vi "Decrement Counter.vi"(5 "Tag Values":string[](array[string]), 7 "Tags":string[](array[string]), 8 "error in (no error)":errorcluster, 9 "Value (1)":i32=1, 10 "Metric Name":string, 11 "StatD Interface in":refnum<class "StatD Interface.lvclass">) -> (0 "error out":errorcluster, 3 "StatD Interface out":refnum<class "StatD Interface.lvclass">)   [LabVIEW 2011, in "StatD Interface.lvclass"]
doc: "Decrement a counter by the amount specified in value (default 1)."
uses:
  StatD Interface.lvclass
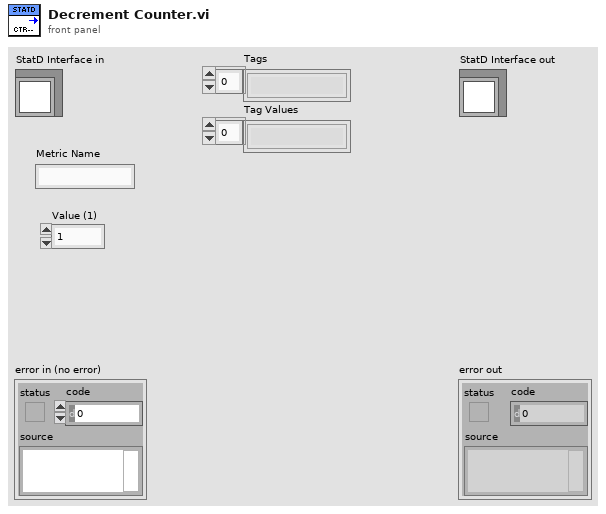
[diagram p1: front panel]
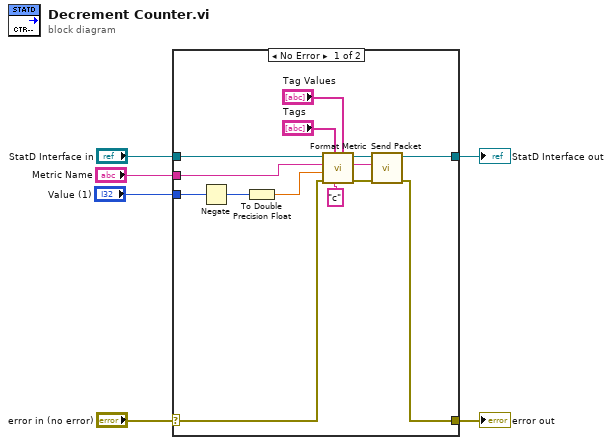
[diagram p0: block diagram]
diagram:
  n1 = case shown="No Error" "error in (no error)" {
    selector: "error in (no error)" -> [w9 w22]
    tunnel: [w19 w22] -> w5
    tunnel: [w20 w21] -> w3
    tunnel: "StatD Interface in" -> [w15 w21]
    tunnel: "Value (1)" -> [w11 _]
    tunnel: "Metric Name" -> [w10 _]
    frame No Error {
      n2 = Negate(x=w11) -> (-x=w7:i32)
      n3 = To Double Precision Float(number=w7) -> (double precision float=w8:dbl)
      n4 = call "Format Metric.vi"("Tag Values"="Tag Values", "Metric Type"="c", "Tags"="Tags", "error in (no error)"=w9, "Metric Value"=w8, "Metric Name"=w10, "StatD Interface in"=w15) -> ("error out"=w17:errorcluster, "Packet"=w16:string, "StatD Interface out"=w18:refnum<class "StatD Interface.lvclass">)  [unwired: 2 in]
      n5 = call "Send Packet.vi"("error in (no error)"=w17, "Packet"=w16, "StatD Interface in"=w18) -> ("error out"=w19:errorcluster, "StatD Interface out"=w20:refnum<class "StatD Interface.lvclass">)  [unwired: 7 in]
    }
    frame Error {
    }
  }
  "error out" <- w5
  "StatD Interface out" <- w3
